vi "Host_DC Power.vi"() -> ()   [LabVIEW 2018]
panel:
  in  "Стоп":bool
  in  "Resource Name":refnum<k15> caption="Первый источник"
  in  "Питание":bool
  in  "Current Limit, мА":dbl
  out "Ток, мА":dbl
  in  "Voltage Level, В":dbl
  out "Waveform Chart":dbl(graph)
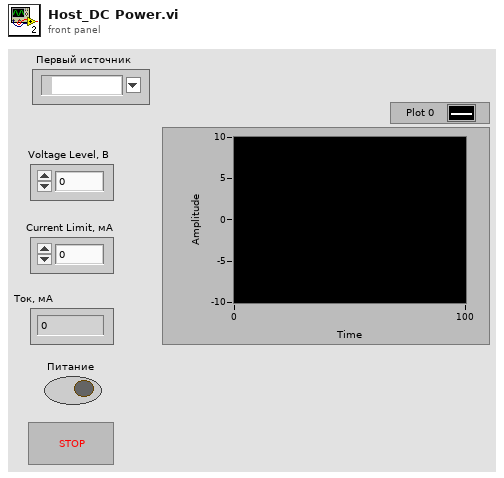
[diagram p1: front panel]
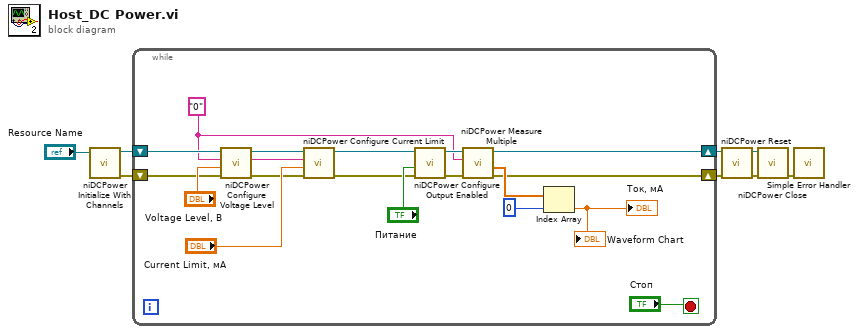
[diagram p0: block diagram]
diagram:
  n1 = call <instrlib>:"niDCPower Initialize With Channels.vi"("resource name"="Resource Name") -> ("error out"=w1:errorcluster, "instrument handle out"=w2:refnum<k15>)  [unwired: 9 in]
  n2 = while {
    shift-right: [w21] -> w8
    shift-left: w2 -> [w14]
    shift-right: [w19] -> w6
    shift-left: w1 -> [w13]
    stop <- "Стоп" stop-if-true
    w12 = "0"
    n3 = call <instrlib>:"niDCPower Configure Voltage Level.vi"("error in (no error)"=w13, "voltage level"="Voltage Level, В", "channel name"=w12, "instrument handle"=w14) -> ("error out"=w20:errorcluster, "instrument handle out"=w22:refnum<k15>)  [unwired: 6 in]
    n4 = call <instrlib>:"niDCPower Configure Current Limit.vi"("error in (no error)"=w20, "current limit"="Current Limit, мА", "channel name"=w12, "instrument handle"=w22) -> ("error out"=w9:errorcluster, "instrument handle out"=w10:refnum<k15>)  [unwired: 6 in]
    n5 = call <instrlib>:"niDCPower Configure Output Enabled.vi"("error in (no error)"=w9, "output enabled"="Питание", "instrument handle"=w10) -> ("error out"=w15:errorcluster, "instrument handle out"=w16:refnum<k15>)  [unwired: 7 in]
    n6 = call <instrlib>:"niDCPower Measure Multiple.vi"("error in (no error)"=w15, "channel name"=w12, "instrument handle"=w16) -> ("error out"=w19:errorcluster, "current measurements"=w24:dbl[], "instrument handle out"=w21:refnum<k15>)  [unwired: 5 in, 1 out]
    n7 = Index Array(array=w24, index=0) -> (element=→"Waveform Chart" →"Ток, мА":dbl)
  }
  n8 = call <instrlib>:"niDCPower Reset.vi"("error in (no error)"=w6, "instrument handle"=w8) -> ("error out"=w5:errorcluster, "instrument handle out"=w7:refnum<k15>)  [unwired: 8 in]
  n9 = call <instrlib>:"niDCPower Close.vi"("error in (no error)"=w5, "instrument handle"=w7) -> ("error out"=w4:errorcluster)  [unwired: 9 in]
  n10 = call <vilib>:"Simple Error Handler.vi"("error in (no error)"=w4) -> ()  [unwired: 4 in, 5 out]
